vi "Delete from Service Map.vi"(8 "error in":errorcluster, 10 "Index":i32, 11 "CAN Task in":refnum<class "CAN Task.lvclass">) -> (0 "error out":errorcluster, 3 "CAN Task out":refnum<class "CAN Task.lvclass">)   [LabVIEW 2024, in "canopen.lvlib" / "CAN Task.lvlib" / "CAN Task.lvclass"]
uses:
  CAN Task.lvclass
  CAN Task.lvclass/CAN Task.ctl
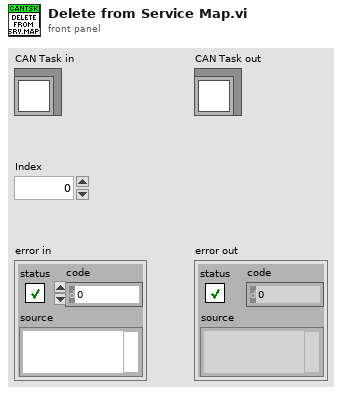
[diagram p1: front panel]
types:
  T1 = cluster{"CobID":u32, "Data offset":u8, "Data size":u8, "Destination":refnum<vi>}[]
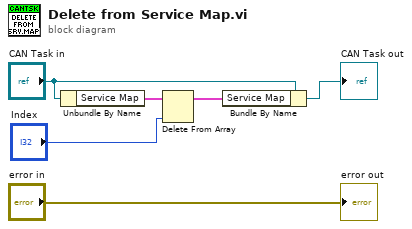
[diagram p0: block diagram]
diagram:
  n1 = Unbundle By Name("CAN Task in") -> ("Service Map"=w5:T1)
  n2 = Delete From Array(array=w5, index="Index") -> (array with subset deleted=w2:T1)  [unwired: 1 in, 1 out]
  n3 = Bundle By Name(cluster="CAN Task in", "Service Map"=w2) -> (→"CAN Task out":refnum<class "CAN Task.lvclass">)
  "error out" <- "error in"
